vi "new Datatype Filter.vi"(10 "datatype":string) -> (2 "datatype filter out":refnum<class "Filter.lvclass">)   [LabVIEW 2016, in "FPGA Resource Manager System Defintion.lvlib" / "Datatype Filter.lvclass"]
uses:
  Datatype Filter.lvclass
  Filter Parent/Filter.lvclass
  C:/github/VeriStand-FPGA-Resource-Manager/Source/Filters/Filter Parent/Filter.lvclass
  Datatype Filter.lvclass/Datatype Filter.ctl
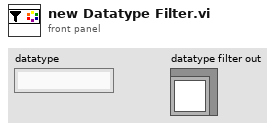
[diagram p1: front panel]
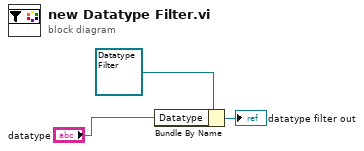
[diagram p0: block diagram]
diagram:
  n1 = Bundle By Name(cluster=refnum<class "Datatype Filter.lvclass"> refnum ("Datatype Filter in"), "Datatype"="datatype") -> (→"datatype filter out":refnum<class "Datatype Filter.lvclass">)
